vi "SimpleCameraGrapImage.vi"(7 "error in (no error)":errorcluster, 10 "Config In":T3 {"Hardware Configuration"."Lasers Configuration"."SettingValues"."785 Power" format="%.1f"; "Hardware Configuration"."Lasers Configuration"."SettingValues"."647 Power" format="%.1f"; "Hardware Configuration"."Lasers Configuration"."SettingValues"."561 Power" format="%.1f"; "Hardware Configuration"."Lasers Configuration"."SettingValues"."532 Power" format="%.1f"; "Hardware Configuration"."Lasers Configuration"."SettingValues"."488 Power" format="%.1f"; "Hardware Configuration"."Lasers Configuration"."SettingValues"."405 Power" format="%.1f"}) -> (0 "error out":errorcluster, 2 "RawImage":T1, 3 "Config Out":T3 {"Hardware Configuration"."Lasers Configuration"."SettingValues"."785 Power" format="%.1f"; "Hardware Configuration"."Lasers Configuration"."SettingValues"."647 Power" format="%.1f"; "Hardware Configuration"."Lasers Configuration"."SettingValues"."561 Power" format="%.1f"; "Hardware Configuration"."Lasers Configuration"."SettingValues"."532 Power" format="%.1f"; "Hardware Configuration"."Lasers Configuration"."SettingValues"."488 Power" format="%.1f"; "Hardware Configuration"."Lasers Configuration"."SettingValues"."405 Power" format="%.1f"})   [LabVIEW 2019]
doc: "Generates sample waveforms according to the signal type in the HW Config input."
uses:
  Settings/Settings.ctl
  HardwareAdapter/Support/Hardware Configuration.ctl
  HardwareAdapter/Support/Camera Configuration.ctl
  D:/SDK/PMQI-LabViewSamples/Examples/Dependencies/PVCamNET.dll
  <vilib>/userdefined/High Color/IMAQdx.ctl
  E:/DevHardSoftware/MMicroscopy/HardwareAdapter/Lasers/Dependencies/Oxxius_Boxx.dll
  HardwareAdapter/Lasers/Dependencies/Oxxius_Boxx.dll
  Logging/Logging Configuration.ctl
  controls/UI Configuration.ctl
  controls/CallBack Refs.ctl
  controls/ImageInfo.ctl
  <vilib>/vision/Image Controls.llb/IMAQ Image.ctl
  <vilib>/numeric/Random Number (Range) U64.vi
  <vilib>/numeric/sub_Random U32.vi
  <vilib>/vision/driver/NI_Vision_Acquisition_Software.lvlib
  Logging/Logging.lvlib
  Settings/Settings.lvlib
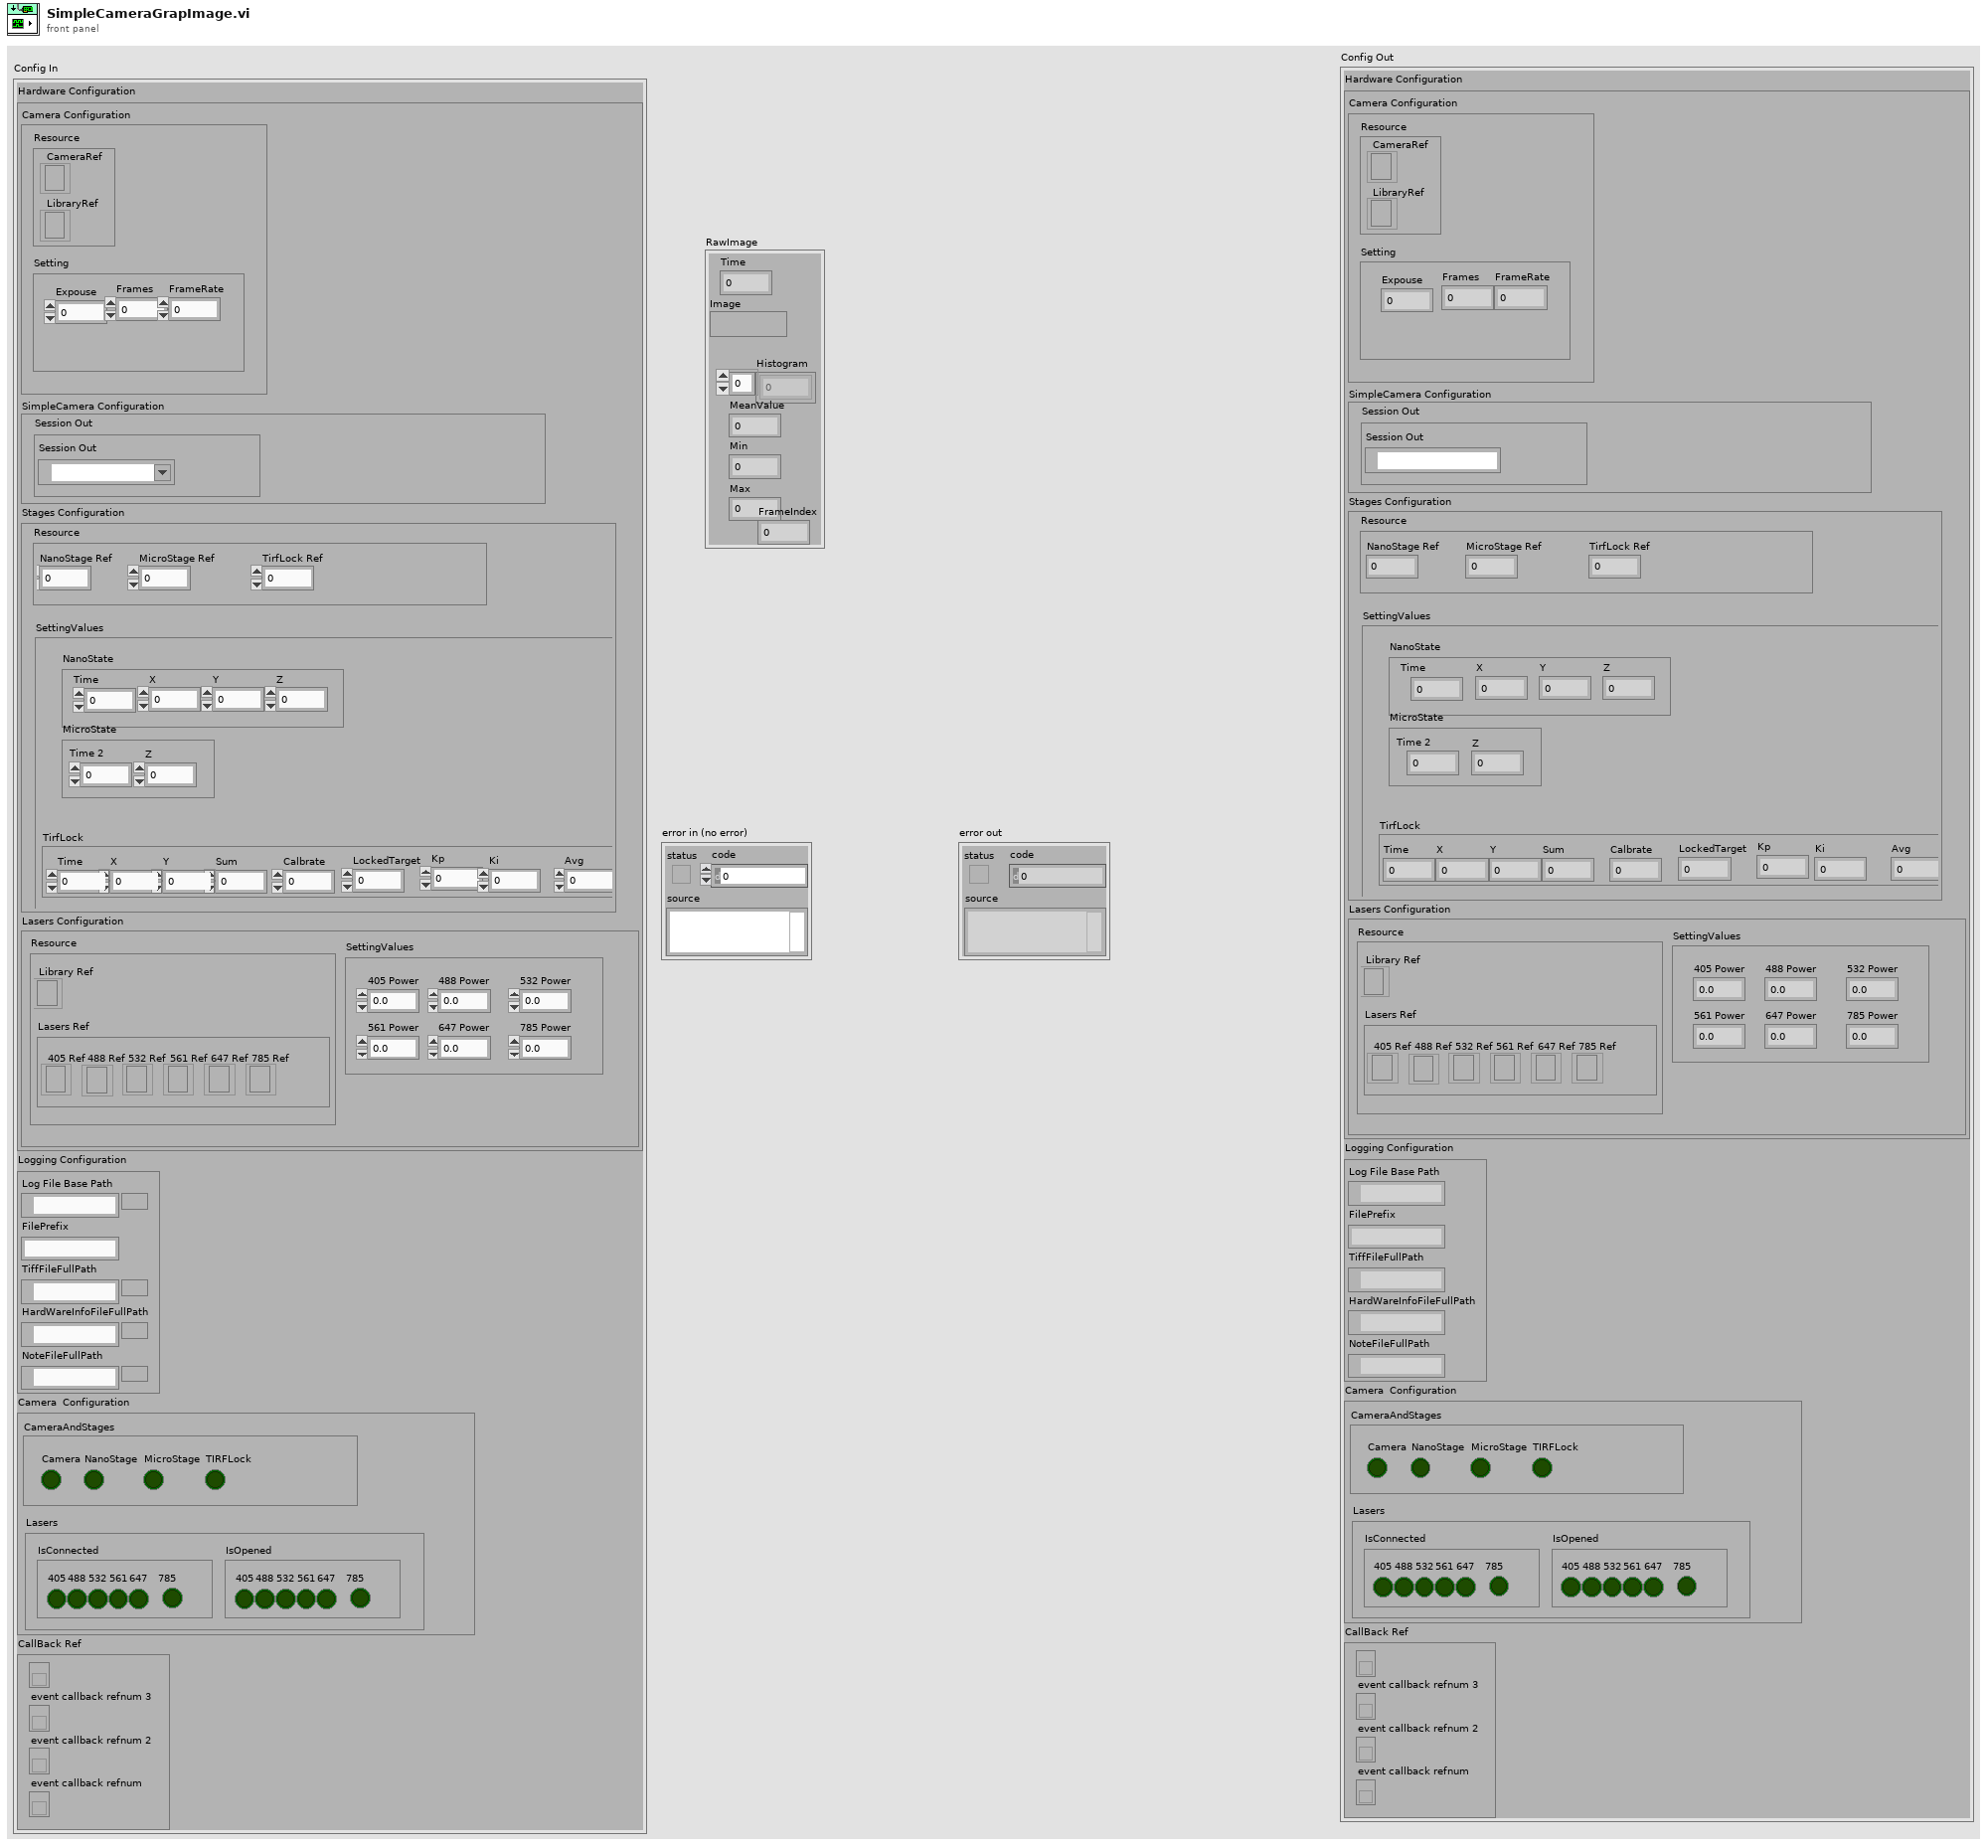
[diagram p1: front panel]
types:
  T1 = typedef "ImageInfo.ctl" = cluster{"Time":dbl, "Image":T2, "Histogram":u32[], "MeanValue":dbl, "Min":u32, "Max":u32, "FrameIndex":dbl}
  T2 = typedef "IMAQ Image.ctl" = refnum<image>
  T3 = typedef "Settings.lvlib/Settings.ctl" = cluster{"Hardware Configuration":T4, "Logging Configuration":T7, "HardWare Status":cluster{"CameraAndStages":T8, "Lasers":cluster{"IsConnected":cluster{"405":bool, "488":bool, "532":bool, "561":bool, "647":bool, "785":bool}, "IsOpened":cluster{"405":bool, "488":bool, "532":bool, "561":bool, "647":bool, "785":bool}}}, "CallBack Ref":T9}
  T4 = typedef "Hardware Configuration.ctl" = cluster{"Camera Configuration":T5, "SimpleCamera Configuration":cluster{"Resource":cluster{"Session Out":T6}}, "Stages Configuration":cluster{"Resource":cluster{"NanoStage Ref":i32, "MicroStage Ref":i32, "TirfLock Ref":i32}, "SettingValues":cluster{"NanoState":cluster{"Time":dbl, "X":dbl, "Y":dbl, "Z":dbl}, "MicroState":cluster{"Time 2":dbl, "Z":dbl}, "TirfLock":cluster{"Time":dbl, "X":dbl, "Y":dbl, "Sum":dbl, "Calbrate":dbl, "LockedTarget":dbl, "Kp":dbl, "Ki":dbl, "Avg":dbl}}}, "Lasers Configuration":cluster{"SettingValues":cluster{"405 Power":sgl, "488 Power":sgl, "532 Power":sgl, "561 Power":sgl, "647 Power":sgl, "785 Power":sgl}, "Resource":cluster{"Library Ref":refnum<k24>, "Lasers Ref":cluster{"405 Ref":refnum<k24>, "488 Ref":refnum<k24>, "532 Ref":refnum<k24>, "561 Ref":refnum<k24>, "647 Ref":refnum<k24>, "785 Ref":refnum<k24>}}}}
  T5 = typedef "Camera Configuration.ctl" = cluster{"Resource":cluster{"CameraRef":refnum<k24>, "LibraryRef":refnum<k24>}, "Setting":cluster{"Expouse":dbl, "Frames":dbl, "FrameRate":dbl}}
  T6 = typedef "IMAQdx.ctl" = refnum<k21>
  T7 = typedef "Logging.lvlib/Logging Configuration.ctl" = cluster{"Log File Base Path":path, "FilePrefix":string, "TiffFileFullPath":path, "HardWareInfoFileFullPath":path, "NoteFileFullPath":path}
  T8 = typedef "UI Configuration.ctl" = cluster{"Camera":bool, "NanoStage":bool, "MicroStage":bool, "TIRFLock":bool}
  T9 = typedef "CallBack Refs.ctl" = cluster{"event callback refnum":refnum<k27>, "event callback refnum 2":refnum<k27>, "event callback refnum 3":refnum<k27>, "event callback refnum 4":refnum<k27>}
  T10 = typedef "Image Type" = u32
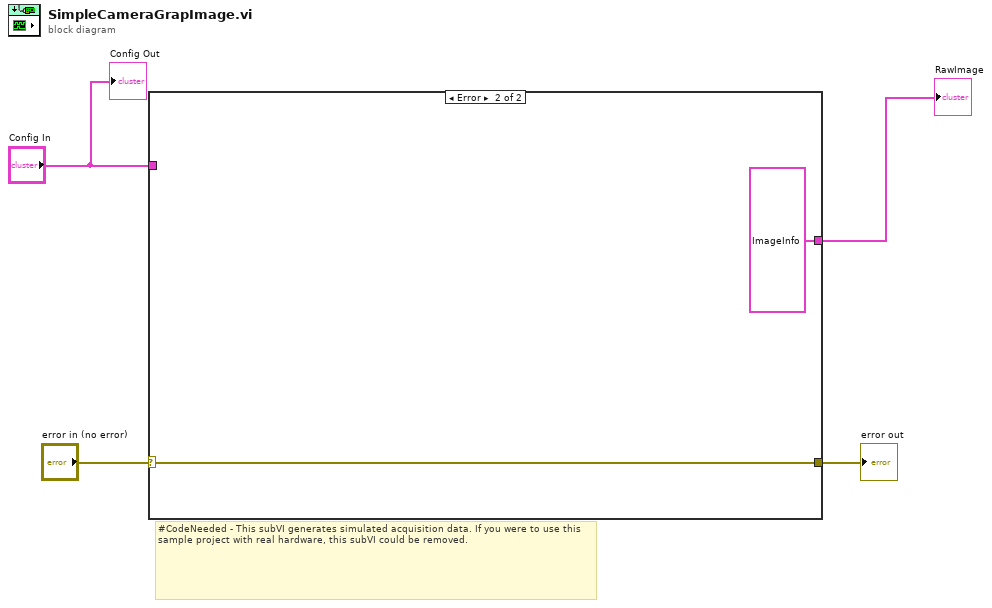
[diagram p0: block diagram]
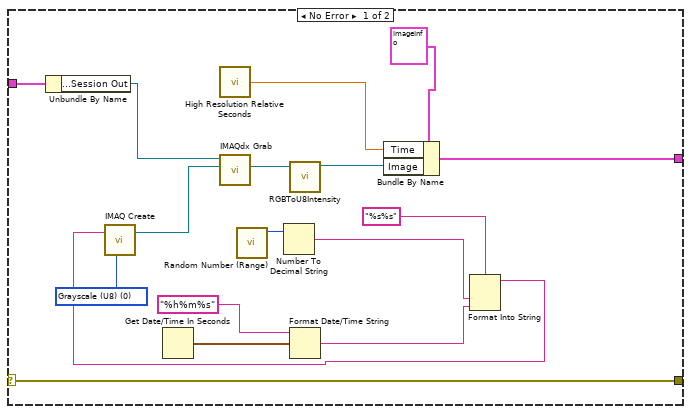
[diagram p2: hidden frame]
diagram:
  # "#CodeNeeded - This subVI generates simulated acquisition data. If you were to use this sample project with real hardware, this subVI could be removed."
  n1 = case shown="Error" "error in (no error)" {
    selector: "error in (no error)" -> [w21 w23]
    tunnel: [w21 w23] -> w3
    tunnel: [w20 T1 {"Time"=0.0, "Image"=refnum, "Histogram"=[], "MeanValue"=0.0, "Min"=0, "Max"=0, "FrameIndex"=0.0} ("RawImage")] -> w1
    tunnel: "Config In" -> [w18 _]
    frame No Error {
      w8 = T10 0 items=["Grayscale (U8)", "Grayscale (I16)", "Grayscale (SGL)", "Complex (CSG)", "RGB (U32)", "HSL (U32)", "RGB (U64)", "Grayscale (U16)"] ("Image Type")
      n2 = Unbundle By Name(w18) -> ("Hardware Configuration.SimpleCamera Configuration.Resource.Session Out"=w17:T6)
      n3 = Get Date/Time In Seconds() -> (seconds since 1Jan1904=w15:timestamp)
      n4 = call <vilib>:"High Resolution Relative Seconds.vi"() -> ("relative seconds"=w19:dbl)
      n5 = call-poly <vilib>:"Random Number (Range).vi"() -> ("number"=w13:u64)  [unwired: 11 in]
      n6 = Number To Decimal String(number=w13) -> (decimal integer string=w12:string)  [unwired: 1 in]
      n7 = Format Date/Time String(time format string (%c)="%h%m%s", seconds (now)=w15) -> (date/time string=w11:string)  [unwired: 1 in]
      n8 = Format Into String(format string="%s%s", w12, w11) -> (resulting string=w9:string)  [unwired: 2 in, 1 out]
      n9 = call "IMAQ Create"("Image Name"=w9, "Image Type"=w8) -> ("New Image"=w16:T2)  [unwired: 2 in, 2 out]
      n10 = call <vilib>:"IMAQdx Grab.vi"("Image In"=w16, "Session In"=w17) -> ("Image Out"=w7:T2)  [unwired: 2 in, 7 out]
      n11 = call "RGBToU8Intensity.vi"("Image Src"=w7) -> ("Image Dst Out"=w6:T2)  [unwired: 10 in]
      n12 = Bundle By Name(cluster=T1 {"Time"=0.0, "Image"=refnum, "Histogram"=[], "MeanValue"=0.0, "Min"=0, "Max"=0, "FrameIndex"=0.0} ("RawImage"), "Time"=w19, "Image"=w6) -> (w20:T1)
    }
    frame Error {
    }
  }
  "error out" <- w3
  "RawImage" <- w1
  "Config Out" <- "Config In"
